vi "L0_Rate_Scan.vi"() -> ()   [LabVIEW 2012]
uses:
  <vilib>/Utility/NIReport.llb/NI_report.lvclass
  <vilib>/Utility/NIReport.llb/HTML/NI_HTML.lvclass
  <instrlib>/Agilent 8000 Series/Public/Configure/Configure Math (Binary Operation).vi
  <instrlib>/Agilent 8000 Series/Agilent 8000 Series.lvlib
panel:
  out "Threshold":i32
  in  "step":i32=10
  in  "Array":i8[](array[numeric])=[0, 1, 2, 3, 4, 5, 6]
  out "Data":string="empty_read_buffer0_2-65@1\r\n0_2-72@0\r\n"
  out "IPR_count":u32
  in  "Instrument VISA":T1={"AWG VISA"="AgilentGenerator1", "Oscilloscope  VISA "="AgilentOsciloscope", "Integration Board IP"="172.16.17.47", "connection ID"=refnum, "report out"=refnum, "report file path"=path "C:/Users/omartinez/Desktop/L0nL1_Results"}
  out "error out":errorcluster
  in  "error in":errorcluster
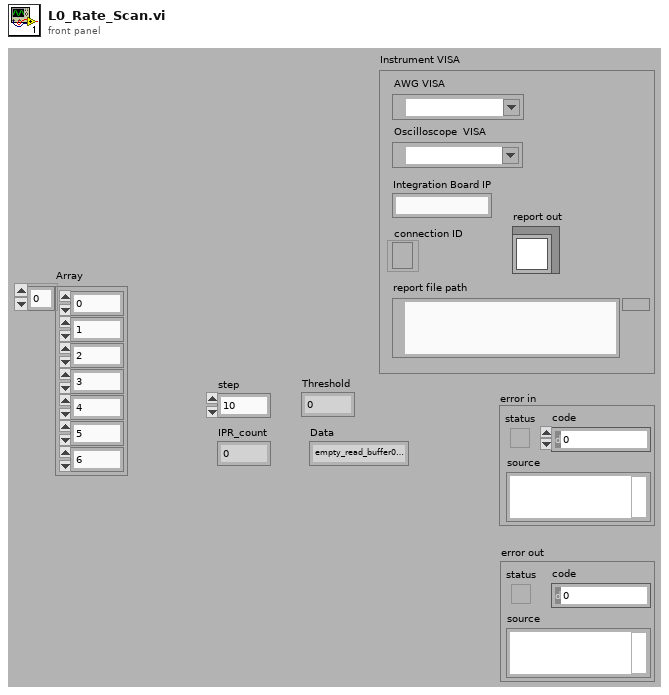
[diagram p1: front panel]
types:
  T1 = cluster{"AWG VISA":refnum<visa-resource-name>, "Oscilloscope  VISA ":refnum<visa-resource-name>, "Integration Board IP":string, "connection ID":refnum<k5>, "report out":refnum<class "NI_report.lvclass">, "report file path":path}
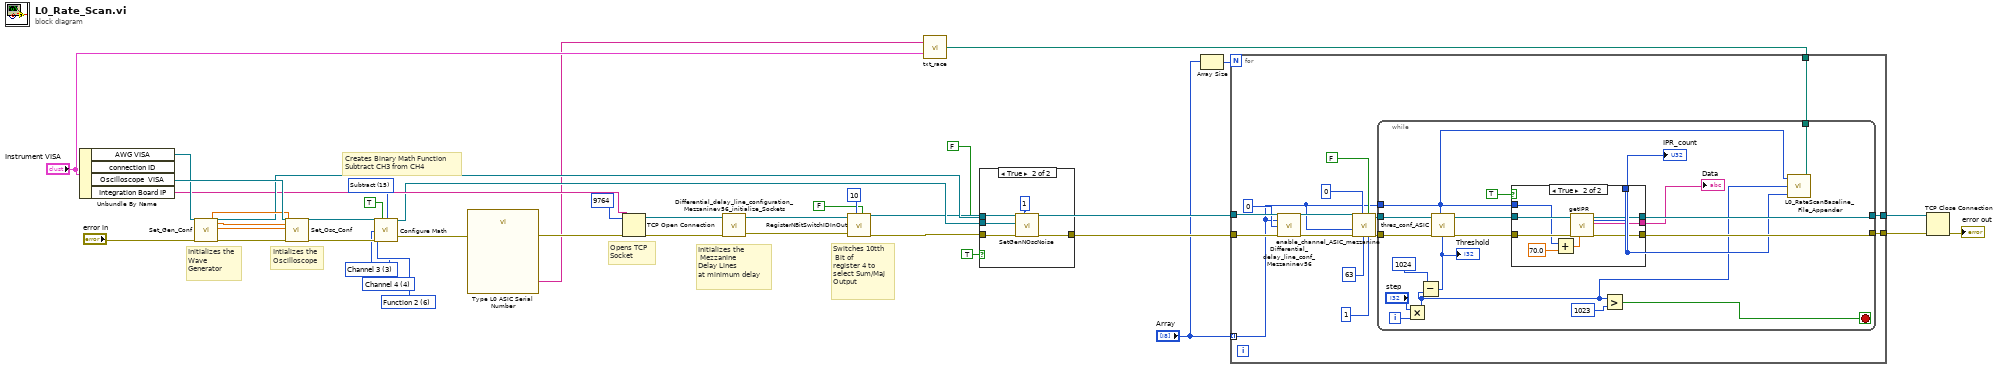
[diagram p0: block diagram]
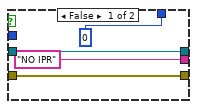
[diagram p2: hidden frame]
diagram:
  w25 = u16 6 items=["Function 1"=5, "Function 2"=6, "Function 3"=7, "Function 4"=8] ("Math Channel (5: Function 1)")
  w26 = u16 15 items=["Add"=12, "Divide"=13, "Multiply"=14, "Subtract"=15, "Common Mode"=16, "Versus"=17] ("Math Operation (12: Add)")
  w20 = 3 items=["Channel 1"=1, "Channel 2"=2, "Channel 3"=3, "Channel 4"=4] ("Channel (1: Channel 1)")
  w21 = 4 items=["Channel 1"=1, "Channel 2"=2, "Channel 3"=3, "Channel 4"=4] ("Channel (1: Channel 1)")
  # "Initializes the\n Mezzanine\nDelay Lines \nat minimum delay"
  # "Switches 10tth \n Bit of\nregister 4 to \nselect Sum/Maj\nOutput"
  # "Opens TCP\nSocket"
  # "Creates Binary Math Function\nSubtract CH3 from CH4"
  # "Intializes the\nOscilloscope"
  # "Initializes the \nWave\nGenerator"
  n1 = Unbundle By Name("Instrument VISA") -> ("AWG VISA"=w35:refnum<visa-resource-name>, "Oscilloscope  VISA"=w36:refnum<visa-resource-name>, "Integration Board IP"=w28:string)  [unwired: 1 out]
  n2 = call "Set_Gen_Conf.vi"("AWG VISA"=w35, "error in (no error)"="error in") -> ("Amplitude 1 OUT"=w33:dbl, "VISA resource name out"=w29:refnum<visa-resource-name>, "Pulse Width in seconds 1 OUT"=w32:dbl, "Trigger Level 1"=w31:dbl, "error out"=w37:errorcluster)  [unwired: 10 in, 3 out]
  n3 = call "Set_Osc_Conf.vi"("VISA resource name"=w36, "Amplitude IN"=w33, "Trigger Level IN"=w31, "Pulse Width in seconds IN"=w32, "error in (no error)"=w37) -> ("VISA resource name out"=w24:refnum<visa-resource-name>, "error out"=w22:errorcluster)  [unwired: 13 in]
  n4 = call-poly <instrlib>:"Configure Math.vi"("VISA resource name"=w24, "Enable Math Channel (T:Enable)"=TRUE, "Math Operation (12: Add)"=w26, "Math Channel (5: Function 1)"=w25, "Math Operand (1: Channel 1)"=w20, "Math Operand (2: Channel 2)"=w21, "error in (no error)"=w22) -> ("VISA resource name out"=w23:refnum<visa-resource-name>, "error out"=w15:errorcluster)  [unwired: 7 in]
  n5 = call "Type L0 ASIC Serial Number"("error in (no error)"=w15) -> ("Serial Number"=w5:string, "error out"=w6:errorcluster)  [unwired: 16 in, 1 out]
  n6 = TCP Open Connection(address=w28, remote port or service name=9764, error in (no error)=w6) -> (connection ID=w12:refnum<k5>, error out=w14:errorcluster)  [unwired: 2 in]
  n7 = call "Differential_delay_line_configuration_Mezzaninev56_initialize_Sockets.vi"("connection ID"=w12, "error in (no error)"=w14) -> ("connection ID out"=w11:refnum<k5>, "error out 2"=w13:errorcluster)  [unwired: 6 in]
  n8 = call "RegisterNBitSwitchIDInOut.vi"("Switch Bit"=FALSE ("Sum/Maj"), "N Bit"=10, "error in (no error)"=w13, "connection ID"=w11) -> ("error out"=w18:errorcluster, "connection ID out"=w17:refnum<k5>)  [unwired: 5 in]
  n9 = call "txt_race.vi"("input cluster"="Instrument VISA", "Serial Number"=w5) -> ("appended path"=w3:path)
  n10 = case shown="True" TRUE {
    tunnel: [w40 w46] -> w9
    tunnel: FALSE ("Gen Active") -> [_ w45]
    tunnel: w23 -> [_ w44]
    tunnel: w29 -> [_ w43]
    tunnel: w18 -> [w40 w42]
    frame False {
    }
    frame True {
      n11 = call "SetGenNOscNoise.vi"("Enable Output"=w45, "NChannels"=1, "error in (no error)"=w42, "VISA resource name"=w44, "AWG VISA"=w43) -> ("error out 2"=w46:errorcluster)  [unwired: 6 in]
    }
  }
  n12 = Array Size(array="Array") -> (size(s)=w2:i32)
  n13 = for {
    N: w2 -> [_]
    tunnel: [w61] -> w30
    tunnel: w17 -> [w60]
    tunnel: [w59] -> w16
    tunnel: w9 -> [w58]
    tunnel: "Array" -> [w48] mode=indexing
    tunnel: w3 -> [w47]
    n14 = call "Differential_delay_line_conf_Mezzaninev56.vi"("connection ID"=w60, "channel"=w48, "Delay value"=0 ("Delay Enable"), "error in (no error)"=w58) -> ("connection ID out"=w56:refnum<k5>, "error out 2"=w57:errorcluster)  [unwired: 4 in, 6 out]
    n15 = call "enable_channel_ASIC_mezzanine.vi"("Clip_sel_b"=1 ("Clipping Select"), "maj/sum"=FALSE, "Ib_clipVb"=63 ("Ib Clip select"), "Att gain"=0 ("Attenuation Select"), "error in"=w57, "Channel"=w48, "connection ID"=w56) -> ("error out"=w52:errorcluster, "connection ID out"=w51:refnum<k5>)  [unwired: 2 in, 1 out]
    n16 = while {
      tunnel: [w79] -> w61
      tunnel: [w78] -> w59
      tunnel: w48 -> [w66]
      tunnel: w52 -> [w74]
      tunnel: w51 -> [w73]
      tunnel: w47 -> [w69]
      i -> [w64]
      stop <- w70 stop-if-true
      n17 = Multiply(x="step", y=w64) -> (x*y=w62:i32)
      n18 = Subtract(x=i16 1024, y=w62) -> (x-y=w67:i32)
      "Threshold" <- w67
      n19 = call "thres_conf_ASIC.vi"("threshold"=w67, "Ring"=w66, "error out 3"=w74, "connection ID"=w73) -> ("error out 2"=w72:errorcluster, "connection ID out"=w75:refnum<k5>)  [unwired: 4 in, 2 out]
      n20 = case shown="True" TRUE ("IPR?") {
        tunnel: w72 -> [w83 w92]
        tunnel: [w83 w85] -> w79
        tunnel: w75 -> [w82 w91]
        tunnel: [w82 w90] -> w78
        tunnel: [u32 0 ("IPR_count") w87] -> w68
        tunnel: ["NO IPR" ("Data") w86] -> w77
        tunnel: w66 -> [_ w84]
        frame False {
        }
        frame True {
          n21 = Add(x=w84, y=70.0) -> (x+y=w89:dbl)
          n22 = call "getIPR.vi"("Address"=w89, "error in"=w92, "connection ID"=w91) -> ("error out"=w85:errorcluster, "Data"=w86:string, "connection ID out"=w90:refnum<k5>, "IPR_count"=w87:u32)  [unwired: 5 in]
        }
      }
      "IPR_count" <- w68
      "Data" <- w77
      n23 = Greater?(x=w62, y=1023 ("x")) -> (0:w70:bool)
      n24 = call "L0_RateScanBaseline_File_Appender.vi"("file path (dialog if empty)"=w69, "IPR"=w68, "Threshold"=w62, "CH"=w66) -> ()
    }
  }
  n25 = TCP Close Connection(connection ID=w16, error in (no error)=w30) -> (error out=→"error out":errorcluster)  [unwired: 1 in, 1 out]
